vi "Add AO Register.vi"(8 "error in (no error)":errorcluster, 9 "Mapping":T1={"DataType"=enum."U16", "Starting Address"=0, "Sub-Index (Bool)"=0, "VS Reference"=0}, 10 "Label":string="Holding Register", 11 "Node Ref In":T3 format="%.0x") -> (0 "error out":errorcluster, 2 "Channel Ref out":T3 format="%.0x", 3 "Node Ref out":T3 format="%.0x")   [LabVIEW 2015, in "Modbus Master System Explorer.lvlib"]
uses:
  Modbus Master System Explorer.lvlib
  <vilib>/NI Veristand/Custom Device API/Custom Device Item Ref.ctl
  Shared/Controls/Data Model/Mapping.ctl
  Shared/Controls/Data Model/DataType.ctl
  <vilib>/NI Veristand/Custom Device API/Custom Device Channel.ctl
  <vilib>/NI Veristand/Custom Device API/Custom Device Channel Type.ctl
  Modbus Type.ctl
  Shared/Constants.vi
  <vilib>/NI VeriStand/Custom Device API/Custom Device API.lvlib
  Shared/Modbus Master Shared.lvlib
  <vilib>/NI VeriStand/Custom Device Tools/Custom Device Utility Library/Custom Device Utility Library.lvlib
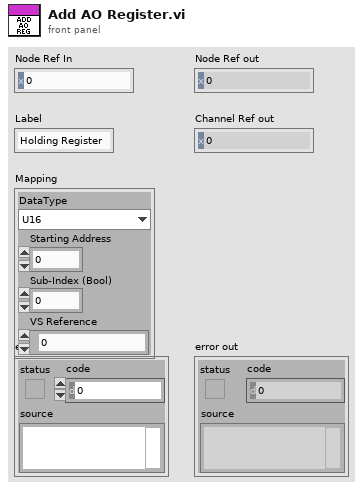
[diagram p1: front panel]
types:
  T1 = typedef "Modbus Master Shared.lvlib/Mapping.ctl" = cluster{"DataType":T2, "Starting Address":u16, "Sub-Index (Bool)":u16, "VS Reference":T3}
  T2 = typedef "Modbus Master Shared.lvlib/DataType.ctl" = enum16{"Double", "Single", "I64", "I32", "I16", "I8", "U64", "U32", "U16", "U8", "Boolean"}
  T3 = typedef "Custom Device API.lvlib/Custom Device Item Ref.ctl" = u64
  T4 = typedef "Custom Device API.lvlib/Custom Device Channel Type.ctl" = enum16{"Input", "Output"}
  T5 = typedef "Modbus Master Shared.lvlib/Modbus Type.ctl" = enum16{"Coil", "Discrete Input", "Holding Register", "Input Register"}
  T6 = typedef "Custom Device API.lvlib/Custom Device Channel.ctl" = cluster{"Type":T4, "Units":string, "Default Value":dbl, "Faultable":bool, "Scalable":bool}
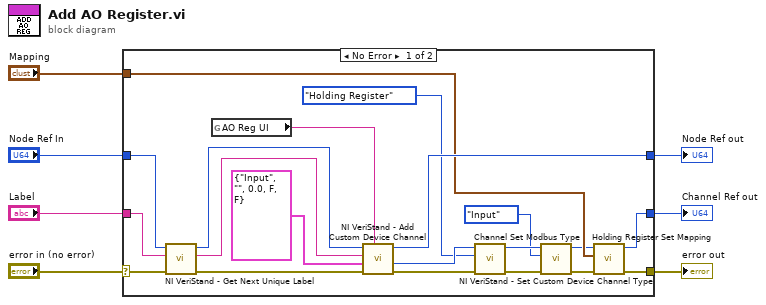
[diagram p0: block diagram]
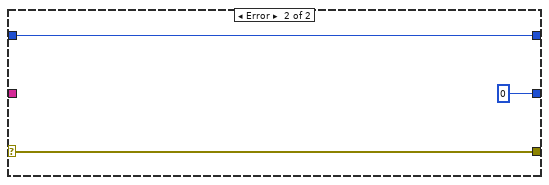
[diagram p2: hidden frame]
diagram:
  n1 = case shown="No Error" "error in (no error)" {
    selector: "error in (no error)" -> [w21 w29]
    tunnel: "Node Ref In" -> [w23 w30]
    tunnel: [w20 w30] -> w5
    tunnel: [w17 w29] -> w4
    tunnel: [w18 T3 0 ("Item Ref out")] -> w3
    tunnel: "Label" -> [w19 _]
    tunnel: "Mapping" -> [w16 _]
    frame No Error {
      n2 = call <vilib>:"NI VeriStand - Get Next Unique Label.vi"("error in (no error)"=w21, "Label"=w19, "Parent Ref in"=w23) -> ("error out"=w25:errorcluster, "Label out"=w26:string, "Parent Ref dup"=w24:T3)  [unwired: 5 in, 1 out]
      n3 = global read "Constants.vi" "AO Reg UI"() -> (w22:string)
      n4 = call <vilib>:"NI VeriStand - Add Custom Device Channel.vi"("GUID (Default Channel)"=w22, "error in (no error)"=w25, "Channel"=T6 {"Type"=enum."Input", "Units"="", "Default Value"=0.0, "Faultable"=FALSE, "Scalable"=FALSE}, "Channel Name"=w26, "Parent Ref in"=w24) -> ("error out"=w14:errorcluster, "Channel Ref"=w15:T3, "Parent Ref out"=w20:T3)  [unwired: 3 in, 1 out]
      n5 = call "Channel Set Modbus Type.vi"("error in (no error)"=w14, "Type"=Modbus_Type."Holding Register", "Channel Ref"=w15) -> ("error out"=w10:errorcluster, "Item Ref out"=w12:T3)  [unwired: 7 in]
      n6 = call <vilib>:"NI VeriStand - Set Custom Device Channel Type.vi"("error in (no error)"=w10, "Type"=Custom_Device_Channel_Type."Input", "Channel Ref in"=w12) -> ("error out"=w9:errorcluster, "Channel Ref out"=w11:T3)  [unwired: 7 in]
      n7 = call "Holding Register Set Mapping.vi"("error in (no error)"=w9, "Mapping"=w16, "Item Ref in"=w11) -> ("error out"=w17:errorcluster, "Item Ref out"=w18:T3)  [unwired: 7 in]
    }
    frame Error {
    }
  }
  "error out" <- w4
  "Node Ref out" <- w5
  "Channel Ref out" <- w3
